vi "log list.vi"(8 "end":string, 9 "start":string, 10 "operaton":string, 11 "worker":i8) -> (2 "log.list":string[][](array[string]))   [LabVIEW 2023]
uses:
  <vilib>/Utility/file.llb/Write Delimited Spreadsheet (string).vi
  <vilib>/Utility/file.llb/Read Delimited Spreadsheet (string).vi
  Shared variables/log.list.vi
  Shared variables/log.lvlib
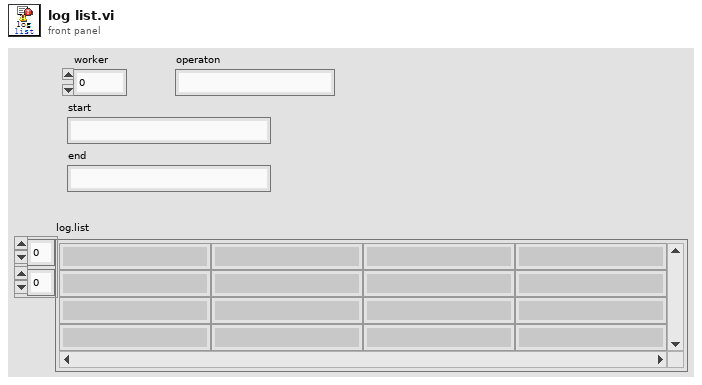
[diagram p1: front panel]
types:
  T1 = enum16{"open", "replace", "create", "open or create", "replace or create", "replace or create with confirmation"}
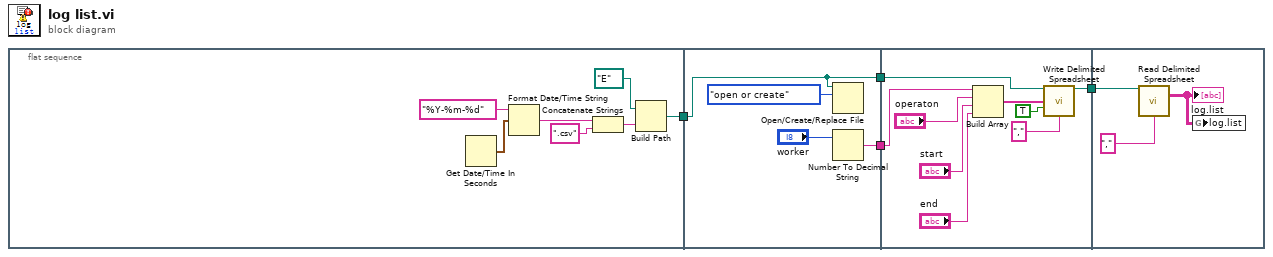
[diagram p0: block diagram]
diagram:
  n1 = flat-sequence {
    tunnel: [w10] -> w4
    tunnel: w4 -> [w15]
    tunnel: [w15] -> w3
    tunnel: [w12] -> w1
    tunnel: w3 -> [w23]
    tunnel: [w20] -> w2
    tunnel: w1 -> [w18]
    tunnel: w2 -> [w27]
    frame #0 {
      n2 = Get Date/Time In Seconds() -> (seconds since 1Jan1904=w8:timestamp)
      n3 = Format Date/Time String(time format string (%c)="%Y-%m-%d", seconds (now)=w8) -> (date/time string=w7:string)  [unwired: 1 in]
      n4 = Concatenate Strings(w7, ".csv" ("string")) -> (w5:string)
      n5 = Build Path(base path=path "E:/", name or relative path=w5) -> (appended path=w10:path)
    }
    frame #1 {
      n6 = Open/Create/Replace File(file path (use dialog)=w15, operation (0:open)=T1."open or create") -> ()  [unwired: 4 in, 3 out]
      n7 = Number To Decimal String(number="worker") -> (decimal integer string=w12:string)  [unwired: 1 in]
    }
    frame #2 {
      n8 = Build Array(w18, "operaton", "start", "end") -> (w19:string[])
      n9 = call-poly <vilib>:"Write Delimited Spreadsheet.vi"("file path (dialog if empty)"=w23, "1D data"=w19, "append to file? (new file:F)"=TRUE, "delimiter (\\t)"="," ("delimiter (\\t)")) -> ("new file path (Not A Path if cancelled)"=w20:path)  [unwired: 10 in, 1 out]
    }
    frame #3 {
      n10 = call-poly <vilib>:"Read Delimited Spreadsheet.vi"("file path (dialog if empty)"=w27, "delimiter (\\t)"="," ("delimiter (\\t)")) -> ("all rows"=w26:string[][])  [unwired: 8 in, 5 out]
      "log.list" <- w26
      n11 = global write "log.list.vi" "log.list"(w26) -> ()
    }
  }
